vi "adsorption_rig_main.vi"() -> ()   [LabVIEW 2020]
uses:
  adam5000_LLB/controls/digital-output-cluster.ctl
  adam5000_LLB/controls/state-enum.ctl
  adam5000_LLB/controls/digitial-input-cluster.ctl
  adam5000_LLB/controls/analog-input-cluster.ctl
  adam5000_LLB/controls/analog-output-cluster.ctl
  adam5000_LLB/controls/thermocouple-input-cluster.ctl
  adam5000_LLB/controls/adam-5000-all-module-datas.ctl
  adam5000_LLB/controls/adam-5000-all-chassis-data.ctl
  adam5000_LLB/controls/adam-5000-chassis-cmd-ack.ctl
  adam5000_LLB/controls/adam-5000-cmd-response.ctl
  adam5000_LLB/controls/adam-5000-chassis-module-types.ctl
  adam5000_LLB/controls/adam-5000-DO-user-input.ctl
  adam5000_LLB/controls/adam-5000-status-indicator-references.ctl
  adam5000_LLB/controls/adam-5000-serial-settings.ctl
  adam5000_LLB/sub-vi/csv-file-logging/filepath-selection.ctl
panel:
  in  "Reset LD":bool
  out "longest delay":u32
  out "Next Log Event mS":u32
  in  "Tab Control":enum32{"System", "Settings"}(tab)
  in  "Flow 4":dbl
  in  "Flow 3":dbl
  in  "Flow 2":dbl
  in  "Flow 1":dbl
  in  "V9: EP1":bool
  in  "V12: EP4":bool
  in  "V10: EP2":bool
  in  "V11: EP3":bool
  in  "V15: \nRecirculation":bool
  in  "V14: HR2":bool
  out "TC9":dbl
  in  "V13: HR1":bool
  out "TC8":dbl
  in  "V8: In4":bool
  out "TC1":dbl
  out "TC2":dbl
  out "TC3":dbl
  out "TC4":dbl
  out "TC5":dbl
  out "TC6":dbl
  out "TC7":dbl
  out "TC10":dbl
  out "TC11":dbl
  out "TC12":dbl
  in  "V1: Ex1":bool
  in  "V2: Ex2":bool
  in  "V4: Ex4":bool
  in  "V5: In1":bool
  in  "V6: In2":bool
  in  "V7: In3":bool
  out "P1: Condenser":dbl
  out "P2: Adsorber 2":dbl
  out "P3: Adsorber 1":dbl
  out "P4: Evaporator":dbl
  in  "V3: Ex3":bool
  in  "Additional CSV Data Heading":string="Flow1,Flow2,Flow3,Flow4"
  in  "Chassis Settings":T1={"VISA resource name"="COM8", "baud rate (19200)"=19200, "Chassis ID"=1}
  in  "Log Filepath Selection":T2={"Log Filepath Source"=enum."Application Relative (Auto)", "Log File Path (Manual)"=path "C:/Users/iwheard/Documents/0000-labview/adam5000-generic-controller/data", "Log File Folder Name"="data", "log file name"="log", "Include Date in Filename"=TRUE, "Include Time in Filename"=TRUE}
  out "Log Filepath":path
  out "log start time":u32
  out "log-elapsed time":dbl format="%.2f"
  in  "CSV Data Headings":string="time (s),T1,T2,T3,T4,T5,T6,T7,T8,T9,T10,T11,T12,P1,P2,P3,P4"
  out "Logged Data String":string
  out "error":errorcluster
  out "Hz":dbl format="%_3g"
  in  "Sample Rate (Hz)":dbl=1.0 min=0.0001 max=4.0 format="%#_4g"
  out "File Open":bool
  out "Logging Active":bool
  out "Error Detected":bool
  in  "Reset":bool
  out "ADAM Connected":bool
  in  "Stop ADAM":bool
  in  "Start Logging":bool
  out "Program State":T3
  in  "Start ADAM":bool
  out "cmd-response":T5
  out "Status Indicators":T6
  in  "Debug Mode":bool
  out "Loop Time (mS)":u32
  out "Loop Counter":i32
  in  "exit":bool
  # "Adsorption Rig 2025"
  # "Built By: \nImogen Heard"
  # "Cold"
  # "Ambient"
  # "Hot"
  # "NV-002"
  # "NV-001"
  # "NV-004"
  # "Flow 4"
  # "Flow 1"
  # "Flow 2"
  # "NV-003"
  # "Flow 3"
  # "Condenser"
  # "Adsorber 1"
  # "Adsorber 2"
  # "Evaporator"
  # "Flow Meter Inputs"
  # "Pressure Sensors"
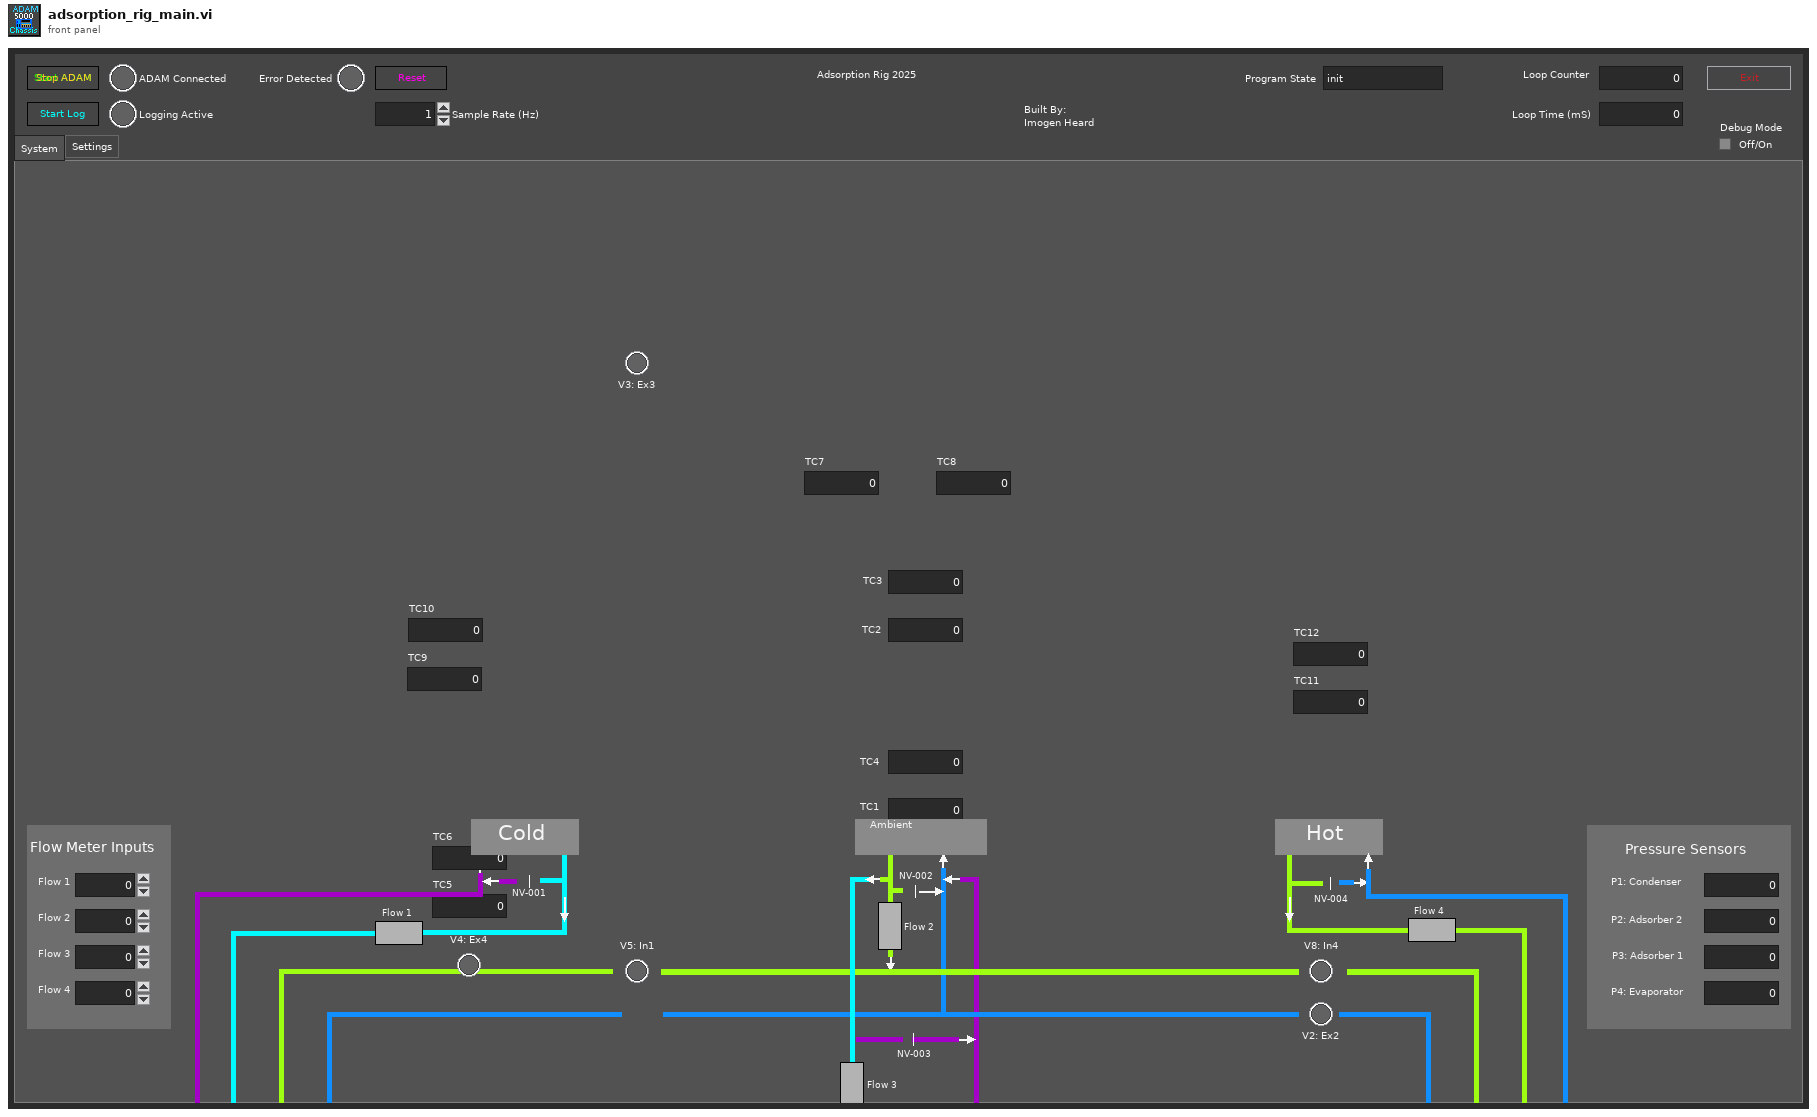
[diagram p1: front panel]
types:
  T1 = typedef "adam-5000-serial-settings.ctl" = cluster{"VISA resource name":refnum<visa-resource-name>, "baud rate (19200)":u32, "Chassis ID":u8}
  T2 = typedef "filepath-selection.ctl" = cluster{"Log Filepath Source":enum16{"Application Relative (Auto)", "VI Relative (Auto)", "Complete Path (Manual)"}, "Log File Path (Manual)":path, "Log File Folder Name":string, "log file name":string, "Include Date in Filename":bool, "Include Time in Filename":bool}
  T3 = typedef "state-enum.ctl" = enum16{"init", "wait", "manual", "start", "run", "reset", "stop", "exit"}
  T4 = typedef "adam-5000-cmd-response.ctl" = cluster{"cmd string":string, "response":string}
  T5 = cluster{"cmd-response:0":T4, "cmd-response:1":T4, "cmd-response:2":T4, "cmd-response:3":T4, "cmd-response:4":T4, "cmd-response:5":T4, "cmd-response:6":T4, "cmd-response:7":T4}
  T6 = cluster{"status-indicator:0":cluster{"Sampling":bool, "Ack":bool}, "status-indicator:1":cluster{"Sampling":bool, "Ack":bool}, "status-indicator:2":cluster{"Sampling":bool, "Ack":bool}, "status-indicator:3":cluster{"Sampling":bool, "Ack":bool}, "status-indicator:4":cluster{"Sampling":bool, "Ack":bool}, "status-indicator:5":cluster{"Sampling":bool, "Ack":bool}, "status-indicator:6":cluster{"Sampling":bool, "Ack":bool}, "status-indicator:7":cluster{"Sampling":bool, "Ack":bool}}
  T7 = enum16{"Digital Output", "Digital Input", "Analog Output", "Analog Input", "Thermocouple", "Power Relay", "empty"}
  T8 = typedef "adam-5000-chassis-module-types.ctl" = cluster{"Slot 0: Module Type":enum16{"Digital Output", "Digital Input", "Analog Output", "Analog Input", "Thermocouple", "Power Relay", "empty"}, "Slot 1: Module Type":enum16{"Digital Output", "Digital Input", "Analog Output", "Analog Input", "Thermocouple", "Power Relay", "empty"}, "Slot 2: Module Type":enum16{"Digital Output", "Digital Input", "Analog Output", "Analog Input", "Thermocouple", "Power Relay", "empty"}, "Slot 3: Module Type":enum16{"Digital Output", "Digital Input", "Analog Output", "Analog Input", "Thermocouple", "Power Relay", "empty"}, "Slot 4: Module Type":enum16{"Digital Output", "Digital Input", "Analog Output", "Analog Input", "Thermocouple", "Power Relay", "empty"}, "Slot 5: Module Type":enum16{"Digital Output", "Digital Input", "Analog Output", "Analog Input", "Thermocouple", "Power Relay", "empty"}, "Slot 6: Module Type":enum16{"Digital Output", "Digital Input", "Analog Output", "Analog Input", "Thermocouple", "Power Relay", "empty"}, "Slot 7: Module Type":enum16{"Digital Output", "Digital Input", "Analog Output", "Analog Input", "Thermocouple", "Power Relay", "empty"}}
  T9 = typedef "adam-5000-chassis-cmd-ack.ctl" = cluster{"cmd-response:0":T4, "cmd-response:1":T4, "cmd-response:2":T4, "cmd-response:3":T4, "cmd-response:4":T4, "cmd-response:5":T4, "cmd-response:6":T4, "cmd-response:7":T4}
  T10 = typedef "adam-5000-all-chassis-data.ctl" = cluster{"slot:0":T11, "slot:1":T11, "slot:2":T11, "slot:3":T11, "slot:4":T11, "slot:5":T11, "slot:6":T11, "slot:7":T11}
  T11 = typedef "adam-5000-all-module-datas.ctl" = cluster{"Digital Outputs":T12, "Digital Inputs":T13, "Analog Outputs":T14, "Analog Inputs":T15, "Thermocouple Inputs (degC)":T16}
  T12 = typedef "digital-output-cluster.ctl" = cluster{"DO0":bool, "DO1":bool, "DO2":bool, "DO3":bool, "DO4":bool, "DO5":bool, "DO6":bool, "DO7":bool}
  T13 = typedef "digitial-input-cluster.ctl" = cluster{"DI0":bool, "DI1":bool, "DI2":bool, "DI3":bool, "DI4":bool, "DI5":bool, "DI6":bool, "DI7":bool}
  T14 = typedef "analog-output-cluster.ctl" = cluster{"AO0":dbl, "AO1":dbl, "AO2":dbl, "AO3":dbl}
  T15 = typedef "analog-input-cluster.ctl" = cluster{"AI0":dbl, "AI1":dbl, "AI2":dbl, "AI3":dbl, "AI4":dbl, "AI5":dbl, "AI6":dbl, "AI7":dbl}
  T16 = typedef "thermocouple-input-cluster.ctl" = cluster{"TC0":dbl, "TC1":dbl, "TC2":dbl, "TC3":dbl, "TC4":dbl, "TC5":dbl, "TC6":dbl}
  T17 = enum8{"Enabled", "Disabled", "Disabled and Grayed Out"}
  T18 = typedef "adam-5000-status-indicator-references.ctl" = cluster{"status-indicator:0":refnum<vi>, "status-indicator:1":refnum<vi>, "status-indicator:2":refnum<vi>, "status-indicator:3":refnum<vi>, "status-indicator:4":refnum<vi>, "status-indicator:5":refnum<vi>, "status-indicator:6":refnum<vi>, "status-indicator:7":refnum<vi>}
  T19 = typedef "adam-5000-DO-user-input.ctl" = cluster{"0:Digital Outputs":T12, "1:Digital Outputs":T12, "2:Digital Outputs":T12, "3:Digital Outputs":T12, "4:Digital Outputs":T12, "5:Digital Outputs":T12, "6:Digital Outputs":T12, "7:Digital Outputs":T12}
  T20 = cluster{"V1: Ex1":bool, "V2: Ex2":bool, "V3: Ex3":bool, "V4: Ex4":bool, "V5: In1":bool, "V6: In2":bool, "V7: In3":bool, "V8: In4":bool}
  T21 = cluster{"V9: EP1":bool, "V10: EP2":bool, "V11: EP3":bool, "V12: EP4":bool, "V13: HR1":bool, "V14: HR2":bool, "V15: \nRecirculation":bool, "V9: EP1":bool}
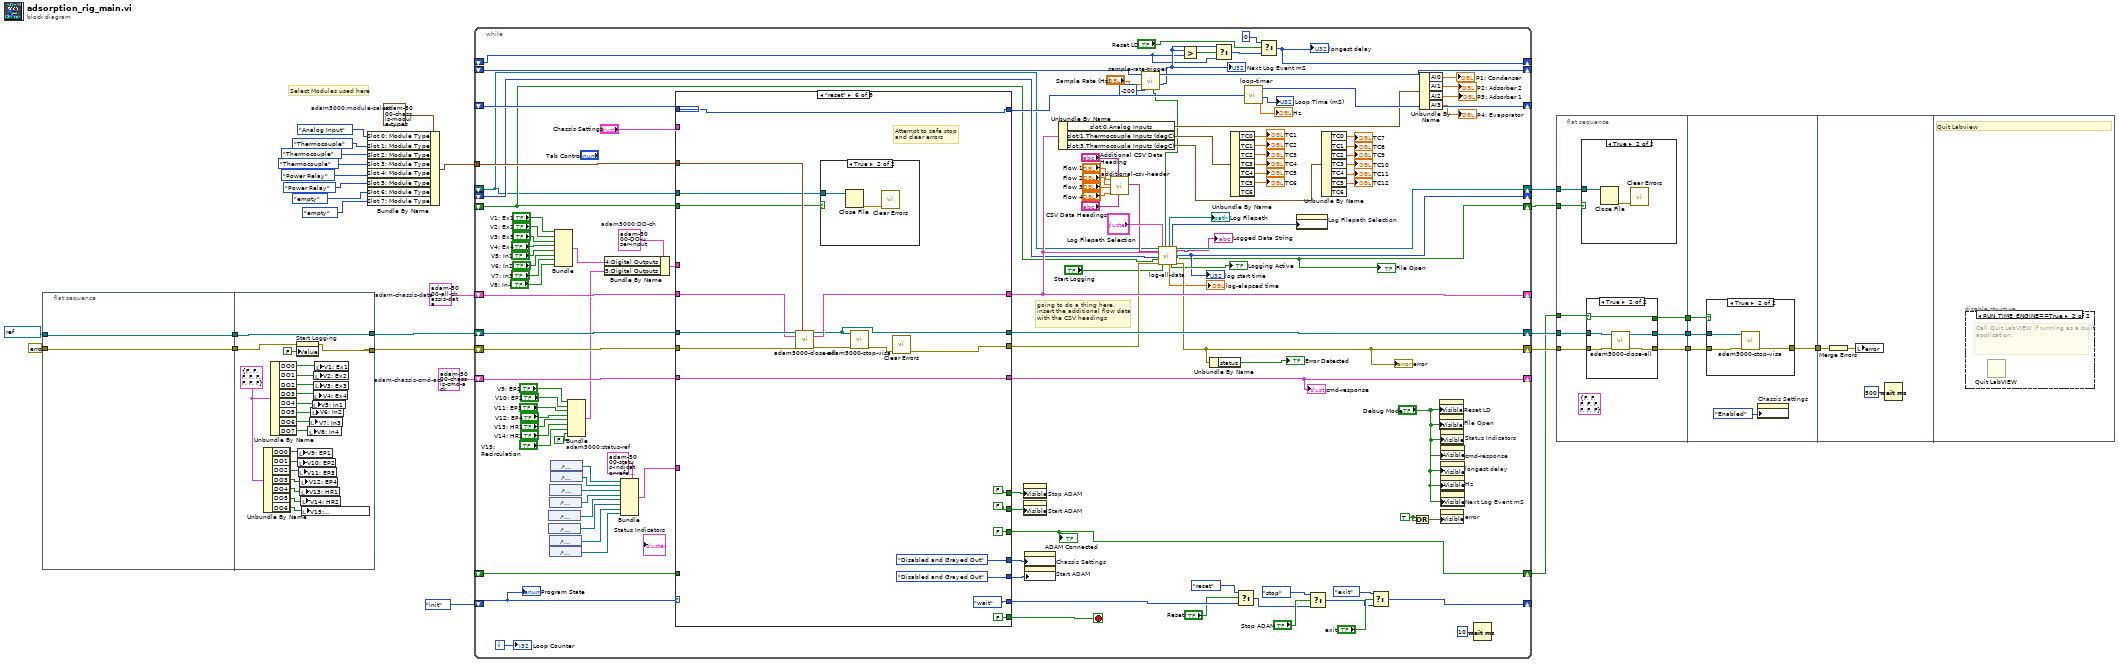
[diagram p0: block diagram]
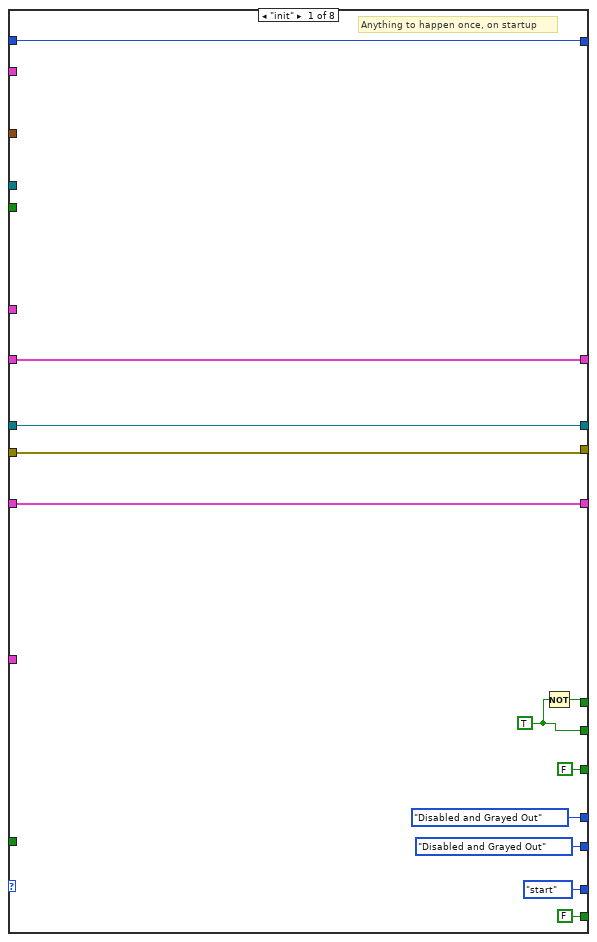
[diagram p6: hidden frame]
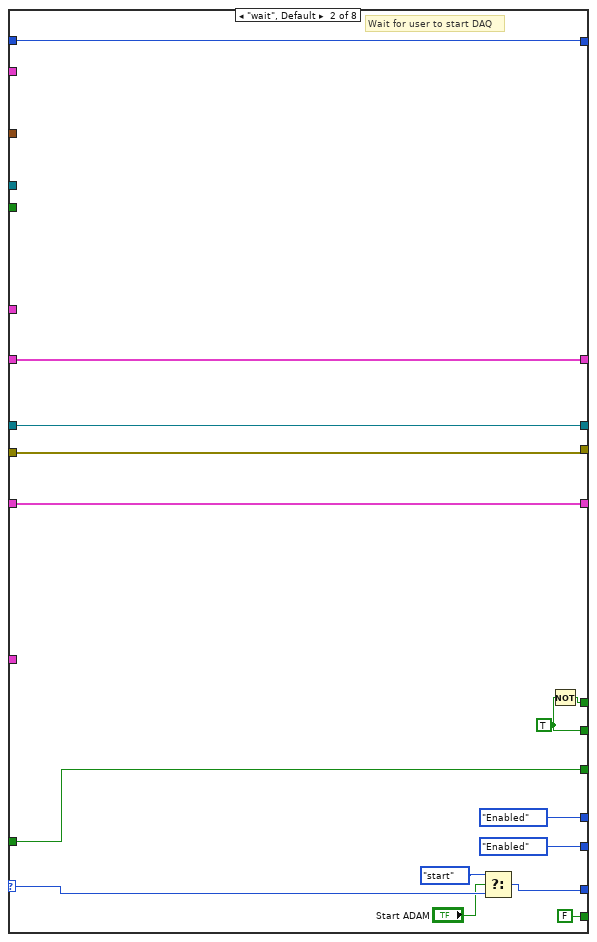
[diagram p7: hidden frame]
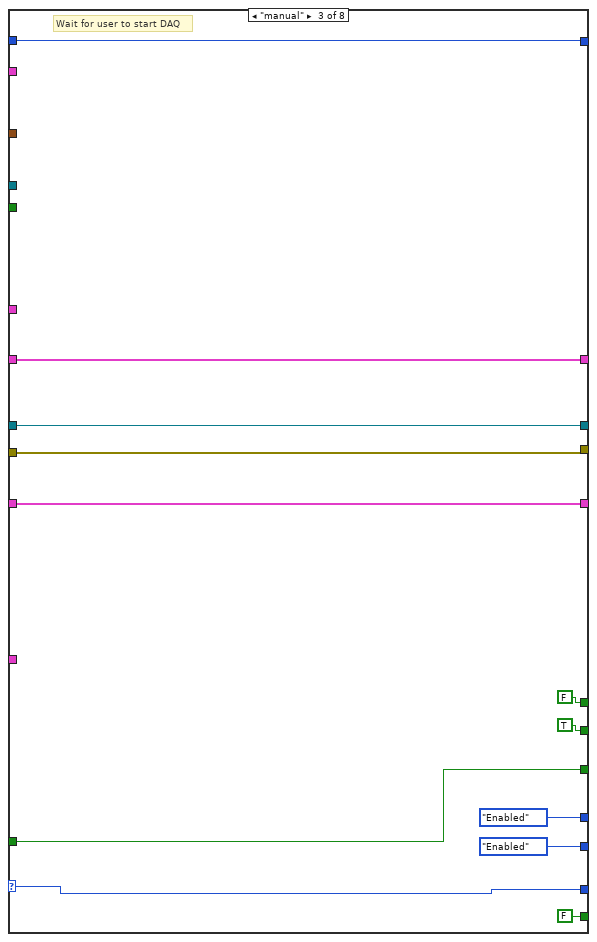
[diagram p8: hidden frame]
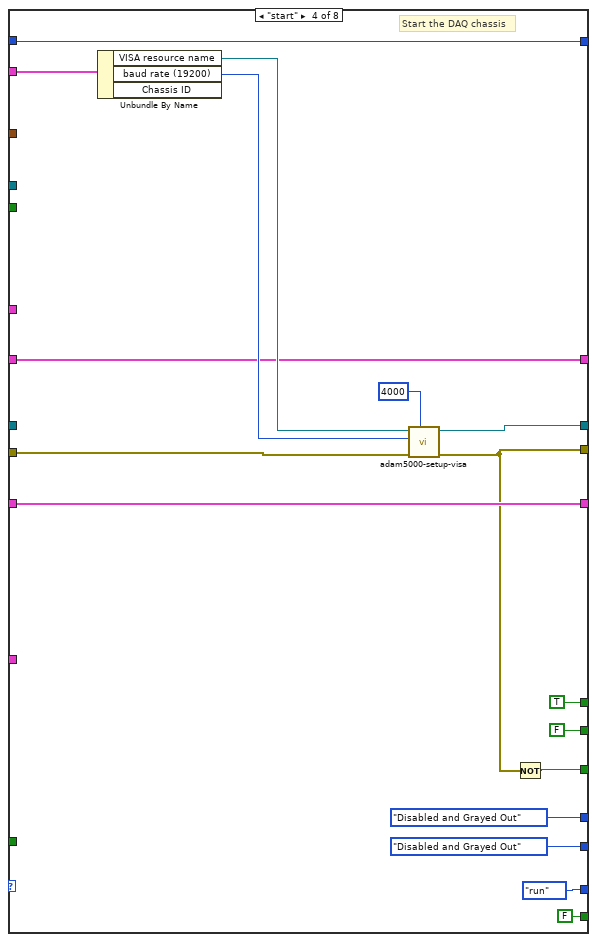
[diagram p9: hidden frame]
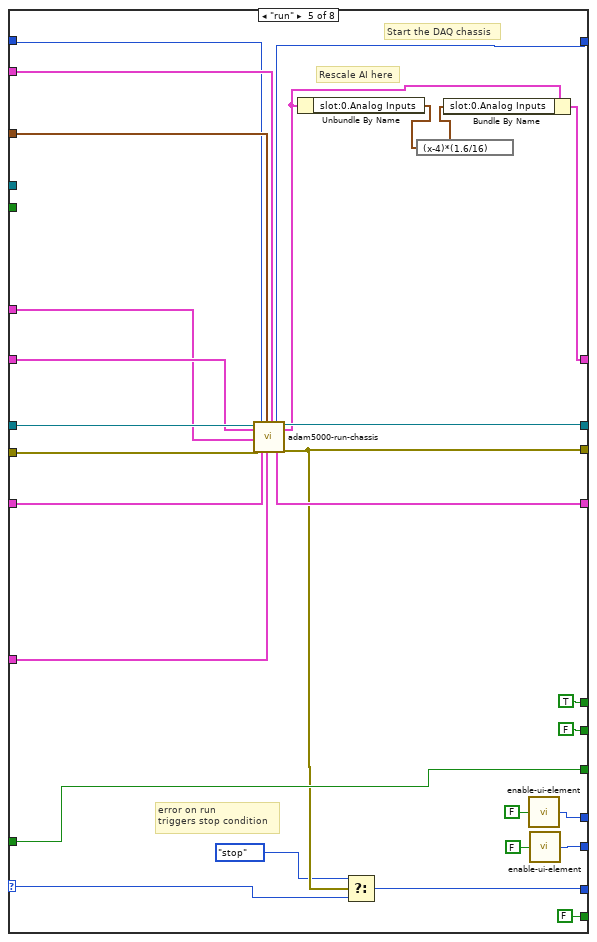
[diagram p10: hidden frame]
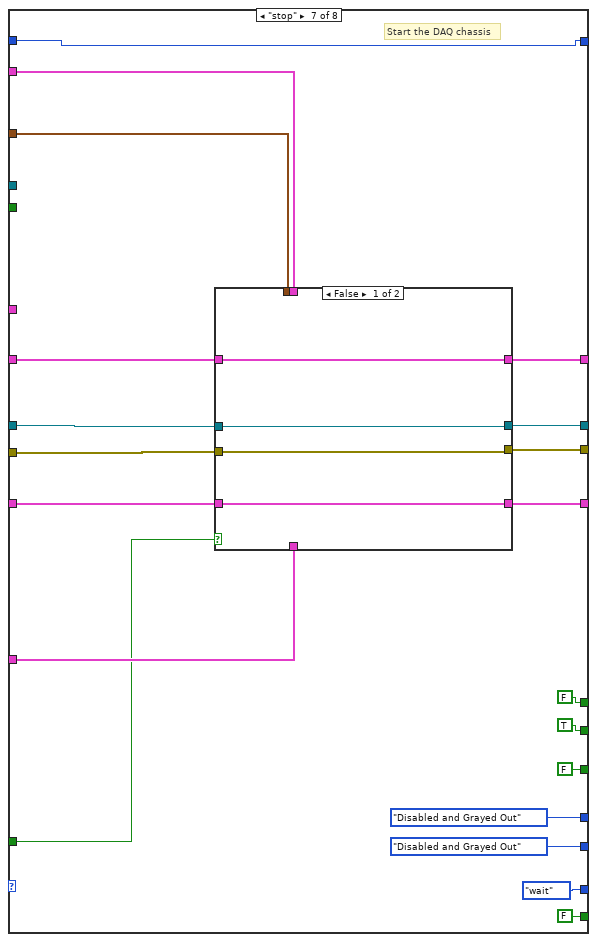
[diagram p12: hidden frame]
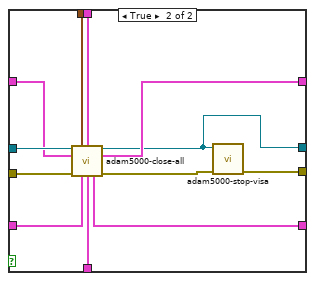
[diagram p13: hidden frame]
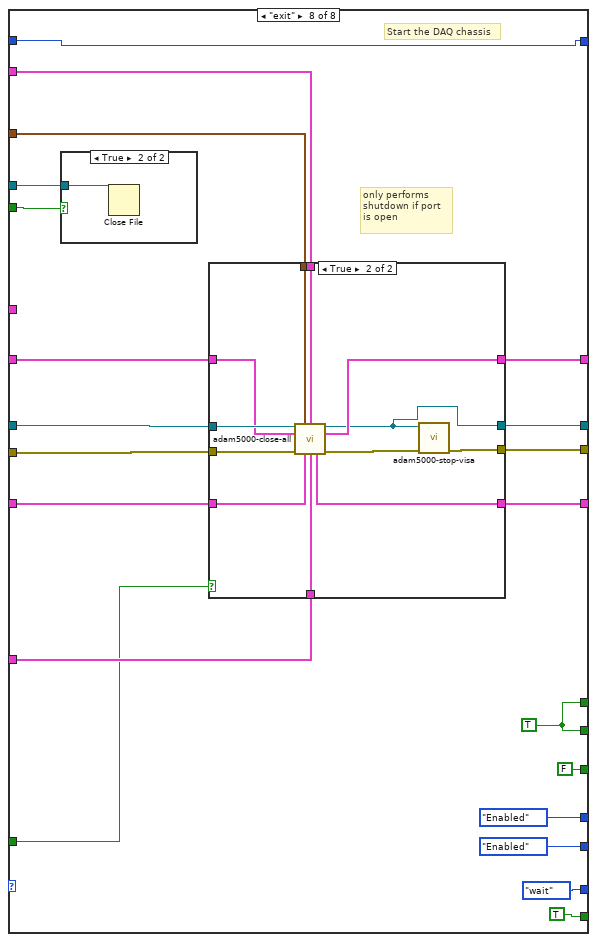
[diagram p14: hidden frame]
diagram:
  w20 = T8 {"Slot 0: Module Type"=enum."Digital Output", "Slot 1: Module Type"=enum."Digital Output", "Slot 2: Module Type"=enum."Digital Output", "Slot 3: Module Type"=enum."Digital Output", "Slot 4: Module Type"=enum."Digital Output", "Slot 5: Module Type"=enum."Digital Output", "Slot 6: Module Type"=enum."Digital Output", "Slot 7: Module Type"=enum."Digital Output"}  # adam5000:module-select
  w25 = T9 {"cmd-response:0"={"cmd string"="", "response"=""}, "cmd-response:1"={"cmd string"="", "response"=""}, "cmd-response:2"={"cmd string"="", "response"=""}, "cmd-response:3"={"cmd string"="", "response"=""}, "cmd-response:4"={"cmd string"="", "response"=""}, "cmd-response:5"={"cmd string"="", "response"=""}, "cmd-response:6"={"cmd string"="", "response"=""}, "cmd-response:7"={"cmd string"="", "response"=""}}  # adam-chassis-cmd-ack
  w26 = T10 {"slot:0"={"Digital Outputs"={"DO0"=FALSE, "DO1"=FALSE, "DO2"=FALSE, "DO3"=FALSE, "DO4"=FALSE, "DO5"=FALSE, "DO6"=FALSE, "DO7"=FALSE}, "Digital Inputs"={"DI0"=FALSE, "DI1"=FALSE, "DI2"=FALSE, "DI3"=FALSE, "DI4"=FALSE, "DI5"=FALSE, "DI6"=FALSE, "DI7"=FALSE}, "Analog Outputs"={"AO0"=0.0, "AO1"=0.0, "AO2"=0.0, "AO3"=0.0}, "Analog Inputs"={"AI0"=0.0, "AI1"=0.0, "AI2"=0.0, "AI3"=0.0, "AI4"=0.0, "AI5"=0.0, "AI6"=0.0, "AI7"=0.0}, "Thermocouple Inputs (degC)"={"TC0"=0.0, "TC1"=0.0, "TC2"=0.0, "TC3"=0.0, "TC4"=0.0, "TC5"=0.0, "TC6"=0.0}}, "slot:1"={"Digital Outputs"={"DO0"=FALSE, "DO1"=FALSE, "DO2"=FALSE, "DO3"=FALSE, "DO4"=FALSE, "DO5"=FALSE, "DO6"=FALSE, "DO7"=FALSE}, "Digital Inputs"={"DI0"=FALSE, "DI1"=FALSE, "DI2"=FALSE, "DI3"=FALSE, "DI4"=FALSE, "DI5"=FALSE, "DI6"=FALSE, "DI7"=FALSE}, "Analog Outputs"={"AO0"=0.0, "AO1"=0.0, "AO2"=0.0, "AO3"=0.0}, "Analog Inputs"={"AI0"=0.0, "AI1"=0.0, "AI2"=0.0, "AI3"=0.0, "AI4"=0.0, "AI5"=0.0, "AI6"=0.0, "AI7"=0.0}, "Thermocouple Inputs (degC)"={"TC0"=0.0, "TC1"=0.0, "TC2"=0.0, "TC3"=0.0, "TC4"=0.0, "TC5"=0.0, "TC6"=0.0}}, "slot:2"={"Digital Outputs"={"DO0"=FALSE, "DO1"=FALSE, "DO2"=FALSE, "DO3"=FALSE, "DO4"=FALSE, "DO5"=FALSE, "DO6"=FALSE, "DO7"=FALSE}, "Digital Inputs"={"DI0"=FALSE, "DI1"=FALSE, "DI2"=FALSE, "DI3"=FALSE, "DI4"=FALSE, "DI5"=FALSE, "DI6"=FALSE, "DI7"=FALSE}, "Analog Outputs"={"AO0"=0.0, "AO1"=0.0, "AO2"=0.0, "AO3"=0.0}, "Analog Inputs"={"AI0"=0.0, "AI1"=0.0, "AI2"=0.0, "AI3"=0.0, "AI4"=0.0, "AI5"=0.0, "AI6"=0.0, "AI7"=0.0}, "Thermocouple Inputs (degC)"={"TC0"=0.0, "TC1"=0.0, "TC2"=0.0, "TC3"=0.0, "TC4"=0.0, "TC5"=0.0, "TC6"=0.0}}, "slot:3"={"Digital Outputs"={"DO0"=FALSE, "DO1"=FALSE, "DO2"=FALSE, "DO3"=FALSE, "DO4"=FALSE, "DO5"=FALSE, "DO6"=FALSE, "DO7"=FALSE}, "Digital Inputs"={"DI0"=FALSE, "DI1"=FALSE, "DI2"=FALSE, "DI3"=FALSE, "DI4"=FALSE, "DI5"=FALSE, "DI6"=FALSE, "DI7"=FALSE}, "Analog Outputs"={"AO0"=0.0, "AO1"=0.0, "AO2"=0.0, "AO3"=0.0}, "Analog Inputs"={"AI0"=0.0, "AI1"=0.0, "AI2"=0.0, "AI3"=0.0, "AI4"=0.0, "AI5"=0.0, "AI6"=0.0, "AI7"=0.0}, "Thermocouple Inputs (degC)"={"TC0"=0.0, "TC1"=0.0, "TC2"=0.0, "TC3"=0.0, "TC4"=0.0, "TC5"=0.0, "TC6"=0.0}}, "slot:4"={"Digital Outputs"={"DO0"=FALSE, "DO1"=FALSE, "DO2"=FALSE, "DO3"=FALSE, "DO4"=FALSE, "DO5"=FALSE, "DO6"=FALSE, "DO7"=FALSE}, "Digital Inputs"={"DI0"=FALSE, "DI1"=FALSE, "DI2"=FALSE, "DI3"=FALSE, "DI4"=FALSE, "DI5"=FALSE, "DI6"=FALSE, "DI7"=FALSE}, "Analog Outputs"={"AO0"=0.0, "AO1"=0.0, "AO2"=0.0, "AO3"=0.0}, "Analog Inputs"={"AI0"=0.0, "AI1"=0.0, "AI2"=0.0, "AI3"=0.0, "AI4"=0.0, "AI5"=0.0, "AI6"=0.0, "AI7"=0.0}, "Thermocouple Inputs (degC)"={"TC0"=0.0, "TC1"=0.0, "TC2"=0.0, "TC3"=0.0, "TC4"=0.0, "TC5"=0.0, "TC6"=0.0}}, "slot:5"={"Digital Outputs"={"DO0"=FALSE, "DO1"=FALSE, "DO2"=FALSE, "DO3"=FALSE, "DO4"=FALSE, "DO5"=FALSE, "DO6"=FALSE, "DO7"=FALSE}, "Digital Inputs"={"DI0"=FALSE, "DI1"=FALSE, "DI2"=FALSE, "DI3"=FALSE, "DI4"=FALSE, "DI5"=FALSE, "DI6"=FALSE, "DI7"=FALSE}, "Analog Outputs"={"AO0"=0.0, "AO1"=0.0, "AO2"=0.0, "AO3"=0.0}, "Analog Inputs"={"AI0"=0.0, "AI1"=0.0, "AI2"=0.0, "AI3"=0.0, "AI4"=0.0, "AI5"=0.0, "AI6"=0.0, "AI7"=0.0}, "Thermocouple Inputs (degC)"={"TC0"=0.0, "TC1"=0.0, "TC2"=0.0, "TC3"=0.0, "TC4"=0.0, "TC5"=0.0, "TC6"=0.0}}, "slot:6"={"Digital Outputs"={"DO0"=FALSE, "DO1"=FALSE, "DO2"=FALSE, "DO3"=FALSE, "DO4"=FALSE, "DO5"=FALSE, "DO6"=FALSE, "DO7"=FALSE}, "Digital Inputs"={"DI0"=FALSE, "DI1"=FALSE, "DI2"=FALSE, "DI3"=FALSE, "DI4"=FALSE, "DI5"=FALSE, "DI6"=FALSE, "DI7"=FALSE}, "Analog Outputs"={"AO0"=0.0, "AO1"=0.0, "AO2"=0.0, "AO3"=0.0}, "Analog Inputs"={"AI0"=0.0, "AI1"=0.0, "AI2"=0.0, "AI3"=0.0, "AI4"=0.0, "AI5"=0.0, "AI6"=0.0, "AI7"=0.0}, "Thermocouple Inputs (degC)"={"TC0"=0.0, "TC1"=0.0, "TC2"=0.0, "TC3"=0.0, "TC4"=0.0, "TC5"=0.0, "TC6"=0.0}}, "slot:7"={"Digital Outputs"={"DO0"=FALSE, "DO1"=FALSE, "DO2"=FALSE, "DO3"=FALSE, "DO4"=FALSE, "DO5"=FALSE, "DO6"=FALSE, "DO7"=FALSE}, "Digital Inputs"={"DI0"=FALSE, "DI1"=FALSE, "DI2"=FALSE, "DI3"=FALSE, "DI4"=FALSE, "DI5"=FALSE, "DI6"=FALSE, "DI7"=FALSE}, "Analog Outputs"={"AO0"=0.0, "AO1"=0.0, "AO2"=0.0, "AO3"=0.0}, "Analog Inputs"={"AI0"=0.0, "AI1"=0.0, "AI2"=0.0, "AI3"=0.0, "AI4"=0.0, "AI5"=0.0, "AI6"=0.0, "AI7"=0.0}, "Thermocouple Inputs (degC)"={"TC0"=0.0, "TC1"=0.0, "TC2"=0.0, "TC3"=0.0, "TC4"=0.0, "TC5"=0.0, "TC6"=0.0}}}  # adam-chassis-data
  # "Select Modules used here"
  n1 = flat-sequence {
    tunnel: errorcluster {"status"=FALSE, "code"=0, "source"=""} ("error in") -> [w29]
    tunnel: refnum<visa-resource-name> "COM8" ("VISA Refnum out") -> [w30]
    tunnel: [w30] -> w2
    tunnel: [w29] -> w1
    tunnel: [w49] -> w9
    tunnel: [w47] -> w7
    tunnel: w2 -> [w49]
    tunnel: w1 -> [w48]
    frame #0 {
    }
    frame #1 {
      w38 = T12 {"DO0"=FALSE, "DO1"=FALSE, "DO2"=FALSE, "DO3"=FALSE, "DO4"=FALSE, "DO5"=FALSE, "DO6"=FALSE, "DO7"=FALSE} ("5:Digital Outputs")
      n2 = Unbundle By Name(w38) -> ("DO0"=w37:bool, "DO1"=w36:bool, "DO2"=w35:bool, "DO3"=w34:bool, "DO4"=w33:bool, "DO5"=w32:bool, "DO6"=w31:bool)
      n3 = Unbundle By Name(w38) -> ("DO0"=w46:bool, "DO1"=w45:bool, "DO2"=w44:bool, "DO3"=w43:bool, "DO4"=w42:bool, "DO5"=w41:bool, "DO6"=w40:bool, "DO7"=w39:bool)
      n4 = property on="Start Logging" class="Bool (strict)"(error in=w48, "Value"=FALSE ("Start Logging")) -> (error out=w47:errorcluster)  [unwired: 1 in, 1 out]
      n5 = local write "V9: EP1"(w37) -> ()
      n6 = local write "V10: EP2"(w36) -> ()
      n7 = local write "V11: EP3"(w35) -> ()
      n8 = local write "V12: EP4"(w34) -> ()
      n9 = local write "V13: HR1"(w33) -> ()
      n10 = local write "V14: HR2"(w32) -> ()
      n11 = local write "V15: \nRecirculation"(w31) -> ()
      n12 = local write "V8: In4"(w39) -> ()
      n13 = local write "V7: In3"(w40) -> ()
      n14 = local write "V6: In2"(w41) -> ()
      n15 = local write "V5: In1"(w42) -> ()
      n16 = local write "V4: Ex4"(w43) -> ()
      n17 = local write "V2: Ex2"(w45) -> ()
      n18 = local write "V3: Ex3"(w44) -> ()
      n19 = local write "V1: Ex1"(w46) -> ()
    }
  }
  n20 = Bundle By Name(cluster=w20, "Slot 0: Module Type"=T7."Analog Input", "Slot 1: Module Type"=T7."Thermocouple", "Slot 2: Module Type"=T7."Thermocouple" ("Slot 1: Module Type"), "Slot 3: Module Type"=T7."Thermocouple" ("Slot 1: Module Type"), "Slot 4: Module Type"=T7."Power Relay" ("Slot 1: Module Type"), "Slot 5: Module Type"=T7."Power Relay" ("Slot 1: Module Type"), "Slot 6: Module Type"=T7."empty" ("Slot 1: Module Type"), "Slot 7: Module Type"=T7."empty" ("Slot 1: Module Type")) -> (w11:T8)
  n21 = while {
    shift-right: [w149] -> _
    shift-left: state-enum."init" ("state-enum") -> [w132]
    shift-right: [w115] -> _
    shift-left: _ -> [w154]
    shift-right: [w141] -> w24
    shift-left: w9 -> [w157]
    shift-right: [w121] -> w23
    shift-left: w7 -> [w156]
    shift-right: [w123] -> _
    shift-left: w26 -> [w153]
    shift-right: [w134] -> _
    shift-left: w25 -> [w151]
    shift-right: [w139] -> w5
    shift-left: _ -> [w140]
    tunnel: w11 -> [w133]
    shift-right: [w111] -> w4
    shift-left: _ -> [w62]
    shift-right: [w112] -> _
    shift-left: _ -> [w122]
    shift-right: [w126] -> w3
    shift-left: _ -> [w61]
    shift-right: [w65] -> _
    shift-left: _ -> [w64]
    shift-right: [w53] -> _
    shift-left: _ -> [w57]
    i -> [w171]
    stop <- w142 stop-if-true
    w160 = T18 {"status-indicator:0"=refnum, "status-indicator:1"=refnum, "status-indicator:2"=refnum, "status-indicator:3"=refnum, "status-indicator:4"=refnum, "status-indicator:5"=refnum, "status-indicator:6"=refnum, "status-indicator:7"=refnum}  # adam5000:status-ref
    w161 = T19 {"0:Digital Outputs"={"DO0"=FALSE, "DO1"=FALSE, "DO2"=FALSE, "DO3"=FALSE, "DO4"=FALSE, "DO5"=FALSE, "DO6"=FALSE, "DO7"=FALSE}, "1:Digital Outputs"={"DO0"=FALSE, "DO1"=FALSE, "DO2"=FALSE, "DO3"=FALSE, "DO4"=FALSE, "DO5"=FALSE, "DO6"=FALSE, "DO7"=FALSE}, "2:Digital Outputs"={"DO0"=FALSE, "DO1"=FALSE, "DO2"=FALSE, "DO3"=FALSE, "DO4"=FALSE, "DO5"=FALSE, "DO6"=FALSE, "DO7"=FALSE}, "3:Digital Outputs"={"DO0"=FALSE, "DO1"=FALSE, "DO2"=FALSE, "DO3"=FALSE, "DO4"=FALSE, "DO5"=FALSE, "DO6"=FALSE, "DO7"=FALSE}, "4:Digital Outputs"={"DO0"=FALSE, "DO1"=FALSE, "DO2"=FALSE, "DO3"=FALSE, "DO4"=FALSE, "DO5"=FALSE, "DO6"=FALSE, "DO7"=FALSE}, "5:Digital Outputs"={"DO0"=FALSE, "DO1"=FALSE, "DO2"=FALSE, "DO3"=FALSE, "DO4"=FALSE, "DO5"=FALSE, "DO6"=FALSE, "DO7"=FALSE}, "6:Digital Outputs"={"DO0"=FALSE, "DO1"=FALSE, "DO2"=FALSE, "DO3"=FALSE, "DO4"=FALSE, "DO5"=FALSE, "DO6"=FALSE, "DO7"=FALSE}, "7:Digital Outputs"={"DO0"=FALSE, "DO1"=FALSE, "DO2"=FALSE, "DO3"=FALSE, "DO4"=FALSE, "DO5"=FALSE, "DO6"=FALSE, "DO7"=FALSE}}  # adam5000:DO-ch
    w143 = TRUE ("Debug Mode")
    # "going to do a thing here,\ninsert the additional flow data \nwith the CSV headings"
    n22 = control-ref of="status-indicator:4"() -> (w165:refnum<vi>)
    n23 = control-ref of="status-indicator:5"() -> (w164:refnum<vi>)
    n24 = control-ref of="status-indicator:3"() -> (w166:refnum<vi>)
    n25 = control-ref of="status-indicator:6"() -> (w163:refnum<vi>)
    n26 = control-ref of="status-indicator:7"() -> (w162:refnum<vi>)
    n27 = control-ref of="status-indicator:2"() -> (w167:refnum<vi>)
    n28 = control-ref of="status-indicator:0"() -> (w169:refnum<vi>)
    n29 = control-ref of="status-indicator:1"() -> (w168:refnum<vi>)
    n30 = Bundle("V1: Ex1"="V1: Ex1", "V2: Ex2"="V2: Ex2", "V3: Ex3"="V3: Ex3", "V4: Ex4"="V4: Ex4", "V5: In1"="V5: In1", "V6: In2"="V6: In2", "V7: In3"="V7: In3", "V8: In4"="V8: In4") -> (w102:T20)  [unwired: 1 in]
    n31 = Bundle("V9: EP1"="V9: EP1", "V10: EP2"="V10: EP2", "V11: EP3"="V11: EP3", "V12: EP4"="V12: EP4", "V13: HR1"="V13: HR1", "V14: HR2"="V14: HR2", "V15: \nRecirculation"="V15: \nRecirculation", "V9: EP1"=FALSE) -> (w93:T21)  [unwired: 1 in]
    n32 = Bundle By Name(cluster=w161, "4:Digital Outputs"=w102, "5:Digital Outputs"=w93) -> (w152:T19)
    n33 = Bundle(cluster=w160, "status-indicator:0"=w169, "status-indicator:1"=w168, "status-indicator:2"=w167, "status-indicator:3"=w166, "status-indicator:4"=w165, "status-indicator:5"=w164, "status-indicator:6"=w163, "status-indicator:7"=w162) -> (w150:T18)
    n34 = case shown="\"reset\"" w132 {
      selector: w132 -> [_ w196 w206 _ w240 _ _ _]
      tunnel: [state-enum."start" ("state-enum") w197 w206 state-enum."run" ("state-enum") w241 state-enum."wait" ("state-enum") state-enum."wait" ("state-enum") state-enum."wait" ("state-enum")] -> w137
      tunnel: [T17."Disabled and Grayed Out" ("Disabled") T17."Enabled" ("Disabled") T17."Enabled" ("Disabled") T17."Disabled and Grayed Out" ("Disabled") w230 T17."Disabled and Grayed Out" ("Disabled") T17."Disabled and Grayed Out" ("Disabled") T17."Enabled" ("Disabled")] -> w159
      tunnel: [T17."Disabled and Grayed Out" ("Disabled") T17."Enabled" ("Disabled") T17."Enabled" ("Disabled") T17."Disabled and Grayed Out" ("Disabled") w228 T17."Disabled and Grayed Out" ("Disabled") T17."Disabled and Grayed Out" ("Disabled") T17."Enabled" ("Disabled")] -> w158
      tunnel: w157 -> [w180 w193 w208 _ w255 w266 w294 w331]
      tunnel: [w180 w193 w208 w225 w253 w260 w284 w319] -> w141
      tunnel: w156 -> [w179 w192 w207 w224 w254 w265 w293 w330]
      tunnel: [w179 w192 w207 w214 w239 w269 w283 w320] -> w120
      tunnel: "Chassis Settings" -> [_ _ _ w223 w252 _ w291 w328]
      tunnel: w133 -> [_ _ _ _ w251 w262 w292 w329]
      tunnel: w154 -> [w178 w190 w205 w218 w250 w271 w285 w322]
      tunnel: [w178 w190 w205 w218 w249 w271 w285 w322] -> w116
      tunnel: w153 -> [w177 w189 w204 w217 w248 w264 w290 w327]
      tunnel: w152 -> [_ _ _ _ w247 _ _ _]
      tunnel: w151 -> [w176 w188 w203 w216 w246 w270 w288 w325]
      tunnel: w150 -> [_ _ _ _ w245 _ w287 w324]
      tunnel: [w176 w188 w203 w216 w244 w270 w286 w323] -> w134
      tunnel: [w177 w189 w204 w217 w234 w263 w289 w326] -> w123
      tunnel: [FALSE FALSE FALSE FALSE FALSE FALSE FALSE TRUE] -> w142
      tunnel: [FALSE w186 w201 w213 w242 FALSE FALSE FALSE] -> w139
      tunnel: w140 -> [_ w186 w201 _ w242 _ w280 w317]
      tunnel: [w173 w184 TRUE ("Visible") FALSE ("Visible") FALSE ("Visible") FALSE ("Visible") TRUE ("Visible") w316] -> w131
      tunnel: [w172 w185 FALSE ("Visible") TRUE ("Visible") TRUE ("Visible") FALSE ("Visible") FALSE ("Visible") w316] -> w130
      tunnel: w62 -> [_ _ _ _ _ w257 _ w314]
      tunnel: w61 -> [_ _ _ _ _ w256 _ w315]
      frame "init" {
        w173 = TRUE ("Visible")
        # "Anything to happen once, on startup"
        n35 = Not(x=w173) -> (.not. x?=w172:bool)
      }
      frame "wait", Default {
        w184 = TRUE ("Visible")
        # "Wait for user to start DAQ"
        n36 = Select(t=state-enum."start" ("state-enum"), s="Start ADAM", f=w196) -> (s? t:f=w197:T3)
        n37 = Not(x=w184) -> (.not. x?=w185:bool)
      }
      frame "manual" {
        # "Wait for user to start DAQ"
      }
      frame "start" {
        # "Start the DAQ chassis"
        n38 = Unbundle By Name(w223) -> ("VISA resource name"=w222:refnum<visa-resource-name>, "baud rate (19200)"=w221:u32)  [unwired: 1 out]
        n39 = call "adam5000-setup-visa.vi"("timeout (10sec)"=u32 4000, "error in"=w224, "baud rate (19200)"=w221, "VISA Refnum in"=w222) -> ("error out"=w214:errorcluster, "VISA Refnum out"=w225:refnum<visa-resource-name>)  [unwired: 6 in]
        n40 = Not(x=w214) -> (.not. x?=w213:bool)
      }
      frame "run" {
        # "Rescale AI here"
        # "error on run\ntriggers stop condition"
        # "Start the DAQ chassis"
        n41 = call "adam5000-run-chassis.vi"("VISA Refnum In"=w255, "adam-chassis-all-data-in"=w248, "adam-chassis-all-DO-in"=w247, "error in"=w254, "loop-time-in"=w250, "adam-chassis-cmd-response-in"=w246, "adam-chassis-module-select-in"=w251, "adam5000:status-ref-in"=w245, "Chassis Settings"=w252) -> ("loop-time-out"=w249:u32, "adam-chassis-cmd-response-out"=w244:T9, "VISA Refnum Out"=w253:refnum<visa-resource-name>, "adam-chassis-all-data-out"=w235:T10, "error out"=w239:errorcluster)  [unwired: 5 in, 1 out]
        n42 = Unbundle By Name(w235) -> ("slot:0.Analog Inputs"=w233:T15)
        n43 = Select(t=state-enum."stop", s=w239, f=w240) -> (s? t:f=w241:T3)
        n44 = expression code="(x-4)*(1.6/16)"(w233) -> (w232:T15)
        n45 = Bundle By Name(cluster=w235, "slot:0.Analog Inputs"=w232) -> (w234:T10)
        n46 = call "enable-ui-element.vi"("Enable UI Element"=FALSE) -> ("UI Element State"=w230:T17)  [unwired: 8 in]
        n47 = call "enable-ui-element.vi"("Enable UI Element"=FALSE) -> ("UI Element State"=w228:T17)  [unwired: 8 in]
      }
      frame "reset" {
        # "Attempt to safe stop\nand clear errors"
        n48 = call "adam5000-close-all.vi"("VISA Refnum in"=w266, "adam5000:module-type-select"=w262, "adam5000:all-data-in"=w264, "error in (no error)"=w265) -> ("VISA Refnum out"=w260:refnum<visa-resource-name>, "adam5000:all-data-out"=w263:T10, "error out"=w267:errorcluster)  [unwired: 8 in, 1 out]
        n49 = case shown="True" w257 {
          tunnel: w256 -> [_ w277]
          frame False {
          }
          frame True {
            n50 = Close File(refnum=w277) -> (error out=w276:errorcluster)  [unwired: 1 in, 1 out]
            n51 = call <vilib>:"Clear Errors.vi"("error in (no error)"=w276) -> ()  [unwired: 5 in, 2 out]
          }
        }
        n52 = call "adam5000-stop-visa.vi"("error in (no error)"=w267, "VISA resource in"=w260) -> ("error out"=w261:errorcluster)  [unwired: 9 in]
        n53 = call <vilib>:"Clear Errors.vi"("error in (no error)"=w261) -> ("error out"=w269:errorcluster)  [unwired: 5 in, 1 out]
      }
      frame "stop" {
        # "Start the DAQ chassis"
        n54 = case shown="False" w280 {
          tunnel: w294 -> [w299 w313]
          tunnel: w293 -> [w298 w312]
          tunnel: w292 -> [_ w311]
          tunnel: w291 -> [_ w310]
          tunnel: w290 -> [w301 w309]
          tunnel: [w301 w308] -> w289
          tunnel: w288 -> [w300 w307]
          tunnel: w287 -> [_ w306]
          tunnel: [w300 w305] -> w286
          tunnel: [w299 w304] -> w284
          tunnel: [w298 w302] -> w283
          frame False {
          }
          frame True {
            n55 = call "adam5000-close-all.vi"("VISA Refnum in"=w313, "adam5000:module-type-select"=w311, "Chassis Settings in"=w310, "adam5000:all-data-in"=w309, "error in (no error)"=w312, "adam-chassis-cmd-ack"=w307, "adam5000:status-ref"=w306) -> ("VISA Refnum out"=w304:refnum<visa-resource-name>, "adam5000:all-data-out"=w308:T10, "adam-chassis-cmd-response-out"=w305:T9, "error out"=w303:errorcluster)  [unwired: 5 in]
            n56 = call "adam5000-stop-visa.vi"("error in (no error)"=w303, "VISA resource in"=w304) -> ("error out"=w302:errorcluster)  [unwired: 9 in]
          }
        }
      }
      frame "exit" {
        w316 = TRUE ("Visible")
        # "only performs\nshutdown if port\nis open"
        # "Start the DAQ chassis"
        n57 = case shown="True" w314 {
          tunnel: w315 -> [_ w335]
          frame False {
          }
          frame True {
            n58 = Close File(refnum=w335) -> ()  [unwired: 1 in, 2 out]
          }
        }
        n59 = case shown="True" w317 {
          tunnel: w331 -> [w338 w351]
          tunnel: w330 -> [w337 w350]
          tunnel: w329 -> [_ w349]
          tunnel: w328 -> [_ w348]
          tunnel: w327 -> [w339 w347]
          tunnel: [w339 w346] -> w326
          tunnel: w325 -> [w336 w345]
          tunnel: w324 -> [_ w344]
          tunnel: [w336 w343] -> w323
          tunnel: [w337 w341] -> w320
          tunnel: [w338 w340] -> w319
          frame False {
          }
          frame True {
            n60 = call "adam5000-close-all.vi"("VISA Refnum in"=w351, "adam5000:module-type-select"=w349, "Chassis Settings in"=w348, "adam5000:all-data-in"=w347, "error in (no error)"=w350, "adam-chassis-cmd-ack"=w345, "adam5000:status-ref"=w344) -> ("VISA Refnum out"=w340:refnum<visa-resource-name>, "adam5000:all-data-out"=w346:T10, "adam-chassis-cmd-response-out"=w343:T9, "error out"=w342:errorcluster)  [unwired: 5 in]
            n61 = call "adam5000-stop-visa.vi"("error in (no error)"=w342, "VISA resource in"=w340) -> ("error out"=w341:errorcluster)  [unwired: 9 in]
          }
        }
      }
    }
    "cmd-response" <- w134
    "ADAM Connected" <- w139
    n62 = property on="Stop ADAM" class="Bool"("Visible"=w130) -> ()  [unwired: 2 in, 2 out]
    n63 = property on="Start ADAM" class="Bool"("Visible"=w131) -> ()  [unwired: 2 in, 2 out]
    n64 = property on="Chassis Settings" class="Clust (strict)"("DisabledEnum"=w159) -> ()  [unwired: 2 in, 2 out]
    n65 = property on="Start ADAM" class="Bool"("DisabledEnum"=w158) -> ()  [unwired: 2 in, 2 out]
    n66 = Unbundle By Name(w123) -> ("slot:0.Analog Inputs"=w85:T15, "slot:1.Thermocouple Inputs (degC)"=w80:T16, "slot:3.Thermocouple Inputs (degC)"=w73:T16)
    n67 = call "additional-csv-header.vi"("CSV Data Headings"="CSV Data Headings", "Additional Text Heading"="Additional CSV Data Heading", "Flow 4"="Flow 4", "Flow 3"="Flow 3", "Flow 2"="Flow 2", "Flow 1"="Flow 1") -> ("new-csv-header"=w86:string)  [unwired: 5 in]
    n68 = call "sample-rate-trigger.vi"("last-event-mS in"=w64, "Sample Rate (Hz)"="Sample Rate (Hz)", "mS modifyer"=-200) -> ("triggered?"=w63:bool, "last-event-mS out"=w65:u32, "Elapsed Time mS"=w58:u32)  [unwired: 4 in, 1 out]
    "Next Log Event mS" <- w58
    n69 = call "log-all-data.vi"("log-file-byte-stream"=w61, "CSV Data Headings"=w86, "adam5000:all-data-in"=w123, "log-start-time(mS)"=w122, "file open?"=w62, "error in (no error)"=w120, "Log Filepath Selection"="Log Filepath Selection", "Start Logging"="Start Logging", "Enable Log Trigger"=w63) -> ("appended path for log file"=→"Log Filepath":path, "log-elapsed time"=→"log-elapsed time":dbl, "log-filepath-enable-state"=w125:T17, "Start Logging"=→"Logging Active":bool, "log-file-bytestream"=w126:refnum<file>, "Logged Data String"=→"Logged Data String":string, "log-start-time(mS)"=w112:u32, "file open?"=w111:bool, "error out"=w121:errorcluster)  [unwired: 2 in]
    "error" <- w121
    "File Open" <- w111
    "log start time" <- w112
    n70 = Greater?(x=w58, y=w57) -> (0:w59:bool)
    n71 = Unbundle By Name(w121) -> ("status"=→"Error Detected":bool)
    n72 = Select(t=w58, s=w59, f=w57) -> (s? t:f=w56:u32)
    n73 = Unbundle By Name(w80) -> ("TC0"=→"TC1":dbl, "TC1"=→"TC2":dbl, "TC2"=→"TC3":dbl, "TC3"=→"TC4":dbl, "TC4"=→"TC5":dbl, "TC5"=→"TC6":dbl)  [unwired: 1 out]
    n74 = Select(t=state-enum."reset", s="Reset", f=w137) -> (s? t:f=w136:T3)
    n75 = call "loop-timer.vi"("loop-time-in"=w116) -> ("Loop Time (mS)"=→"Loop Time (mS)":u32, "loop-time-out"=w115:u32, "Hz"=→"Hz":dbl)  [unwired: 8 in]
    n76 = Select(t=u32 0, s="Reset LD", f=w56) -> (s? t:f=w53:u32)
    "longest delay" <- w53
    n77 = property on="Log Filepath Selection" class="Clust (strict)"("DisabledEnum"=w125) -> ()  [unwired: 2 in, 2 out]
    n78 = Select(t=state-enum."stop", s="Stop ADAM", f=w136) -> (s? t:f=w146:T3)
    n79 = Unbundle By Name(w73) -> ("TC0"=→"TC7":dbl, "TC1"=→"TC8":dbl, "TC2"=→"TC9":dbl, "TC3"=→"TC10":dbl, "TC4"=→"TC11":dbl, "TC5"=→"TC12":dbl)  [unwired: 1 out]
    n80 = Select(t=state-enum."exit", s="exit", f=w146) -> (s? t:f=w149:T3)
    n81 = Or(x=w143, y=w143) -> (x .or. y?=w170:bool)
    n82 = Unbundle By Name(w85) -> ("AI0"=→"P1: Condenser":dbl, "AI1"=→"P2: Adsorber 2":dbl, "AI2"=→"P3: Adsorber 1":dbl, "AI3"=→"P4: Evaporator":dbl)
    n83 = property on="Reset LD" class="Bool"("Visible"="Debug Mode") -> ()  [unwired: 2 in, 2 out]
    n84 = property on="File Open" class="Bool (strict)"("Visible"="Debug Mode") -> ()  [unwired: 2 in, 2 out]
    n85 = property on="Status Indicators" class="Clust (strict)"("Visible"="Debug Mode") -> ()  [unwired: 2 in, 2 out]
    n86 = property on="error" class="Clust (strict)"("Visible"=w170) -> ()  [unwired: 2 in, 2 out]
    n87 = property on="cmd-response" class="Clust (strict)"("Visible"="Debug Mode") -> ()  [unwired: 2 in, 2 out]
    n88 = property on="longest delay" class="DigNum (strict)"("Visible"="Debug Mode") -> ()  [unwired: 2 in, 2 out]
    n89 = property on="Hz" class="DigNum (strict)"("Visible"="Debug Mode") -> ()  [unwired: 2 in, 2 out]
    n90 = property on="Next Log Event mS" class="DigNum (strict)"("Visible"="Debug Mode") -> ()  [unwired: 2 in, 2 out]
    n91 = Wait (ms)(milliseconds to wait=u32 10) -> ()  [unwired: 1 out]
    "Loop Counter" <- w171
    "Program State" <- w132
  }
  n92 = flat-sequence {
    tunnel: w24 -> [w359]
    tunnel: w23 -> [w358]
    tunnel: [w357] -> w22
    tunnel: [w356] -> w21
    tunnel: w5 -> [w355]
    tunnel: [w354] -> w6
    tunnel: w4 -> [w353]
    tunnel: w3 -> [w352]
    tunnel: [w374] -> w27
    tunnel: w22 -> [w373]
    tunnel: w21 -> [w372]
    tunnel: w6 -> [w370]
    tunnel: w27 -> [w380]
    frame #0 {
      (unwired) T12 {"DO0"=FALSE, "DO1"=FALSE, "DO2"=FALSE, "DO3"=FALSE, "DO4"=FALSE, "DO5"=FALSE, "DO6"=FALSE, "DO7"=FALSE} ("5:Digital Outputs")
      n93 = case shown="True" w353 {
        tunnel: w352 -> [_ w361]
        frame False {
        }
        frame True {
          n94 = Close File(refnum=w361) -> (error out=w360:errorcluster)  [unwired: 1 in, 1 out]
          n95 = call <vilib>:"Clear Errors.vi"("error in (no error)"=w360) -> ()  [unwired: 5 in, 2 out]
        }
      }
      n96 = case shown="True" w355 {
        selector: w355 -> [w362 w365]
        tunnel: w359 -> [w364 w369]
        tunnel: w358 -> [w363 w368]
        tunnel: [w363 w367] -> w357
        tunnel: [w364 w366] -> w356
        tunnel: [w362 w365] -> w354
        frame False {
        }
        frame True {
          n97 = call "adam5000-close-all.vi"("VISA Refnum in"=w369, "error in (no error)"=w368) -> ("VISA Refnum out"=w366:refnum<visa-resource-name>, "error out"=w367:errorcluster)  [unwired: 10 in, 2 out]
        }
      }
    }
    frame #1 {
      n98 = case shown="True" w370 {
        tunnel: [w375 w378] -> w374
        tunnel: w373 -> [w375 w377]
        tunnel: w372 -> [_ w376]
        frame False {
        }
        frame True {
          n99 = call "adam5000-stop-visa.vi"("error in (no error)"=w377, "VISA resource in"=w376) -> ("error out"=w378:errorcluster)  [unwired: 9 in]
        }
      }
      n100 = property on="Chassis Settings" class="Clust (strict)"("DisabledEnum"=T17."Enabled" ("Disabled")) -> ()  [unwired: 2 in, 2 out]
    }
    frame #2 {
      n101 = Merge Errors(w380) -> (w379:errorcluster)
      n102 = local write "error"(w379) -> ()
      n103 = Wait (ms)(milliseconds to wait=u32 500) -> ()  [unwired: 1 out]
    }
    frame #3 {
      # "Quit Labview"
      n104 = disable-structure "Conditional Disable Structure" shown="RUN_TIME_ENGINE==True" {
        frame condition #0 (active) {
        }
        frame condition #1 {
          # "Call Quit LabVIEW if running as a built application."
          n105 = Quit LabVIEW() -> ()  [unwired: 1 in]
        }
      }
    }
  }
